vi "Launcher.vi"(8 "error in (no error)":errorcluster, 10 "Log Class":refnum<class "Build_Javier_Lopez_lib_Configuration_Filejson class.lvclass">, 11 "Module Database Manager in":refnum<class "Database Manager.lvclass">) -> (0 "error out":errorcluster)   [LabVIEW 2021, in "Database Manager.lvclass"]
uses:
  Database Manager.lvclass
  <vilib>/Javier Lopez/Configuration File/Json Element/Build_Javier_Lopez_lib_Configuration_Filejson class.lvclass
  Libraries/Database Manager/Database Manager.lvlib
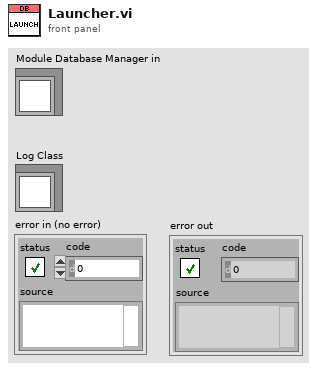
[diagram p1: front panel]
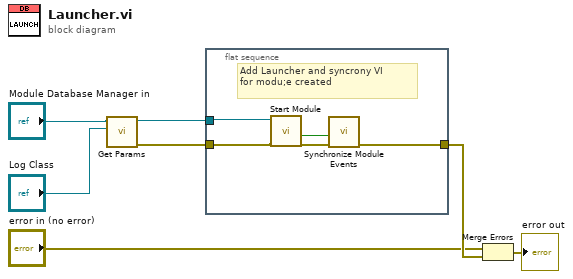
[diagram p0: block diagram]
diagram:
  n1 = call-dynamic "Get Params.vi"("Log Class"="Log Class", "Module Database Manager in"="Module Database Manager in") -> ("error out"=w6:errorcluster, "Module Database Manager out"=w5:refnum<class "Database Manager.lvclass">)  [unwired: 8 in]
  n2 = flat-sequence {
    tunnel: w5 -> [w8]
    tunnel: w6 -> [w10]
    tunnel: [w9] -> w7
    frame #0 {
      # "Add Launcher and syncrony VI\nfor modu;e created"
      n3 = call "Start Module.vi"("error in"=w10, "Database Manager in"=w8) -> ("error out"=w11:errorcluster, "Wait for Event Sync?"=w12:bool)  [unwired: 5 in, 3 out]
      n4 = call "Synchronize Module Events.vi"("error in"=w11, "Wait for Event Sync?"=w12) -> ("error out"=w9:errorcluster)  [unwired: 9 in]
    }
  }
  n5 = Merge Errors("error in (no error)", w7) -> (→"error out":errorcluster)
